vi "TDMS_Create.vi"(0 "reference in":refnum<class "TDMS.lvclass">, 5 "error in (no error)":errorcluster, 6 "Time Data":refnum<class "GSwFormDSP.lvclass">, 7 "Application Name":string, 9 "State Queue":string[](array[string])) -> (14 "reference out":refnum<class "TDMS.lvclass">, 19 "error out":errorcluster)   [LabVIEW 2022 SP3, in "TDMS.lvclass"]
doc: "Constructor."
uses:
  TDMS.lvclass
  C:/Program Files/National Instruments/LabVIEW 2022/vi.lib/addons/_AddQ/G#Object/G#Object.lvclass
  W:/projects/archives/23 Charette AI Group/SPWB/API/Generic Utilities_class/Generic Utilities.lvclass
  API/GSwFormDSP_class/GSwFormDSP.lvclass
  <vilib>/addons/_AddQ/G#Object/G#Object.lvclass
  API/Generic Utilities_class/Generic Utilities.lvclass
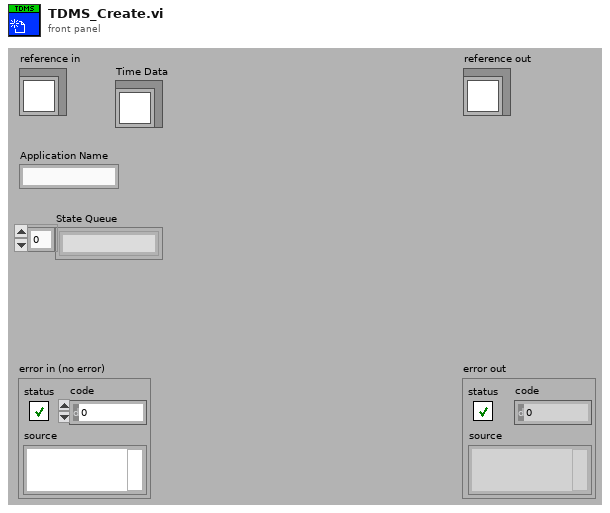
[diagram p1: front panel]
types:
  T1 = typedef "TDMS.lvclass/ObjectAttributesRef.ctl" = refnum<data-value>
  T2 = typedef "TDMS.lvclass/ObjectAttributes.ctl" = cluster{"Time Data":refnum<class "GSwFormDSP.lvclass">, "New Time Data Obj?":bool}
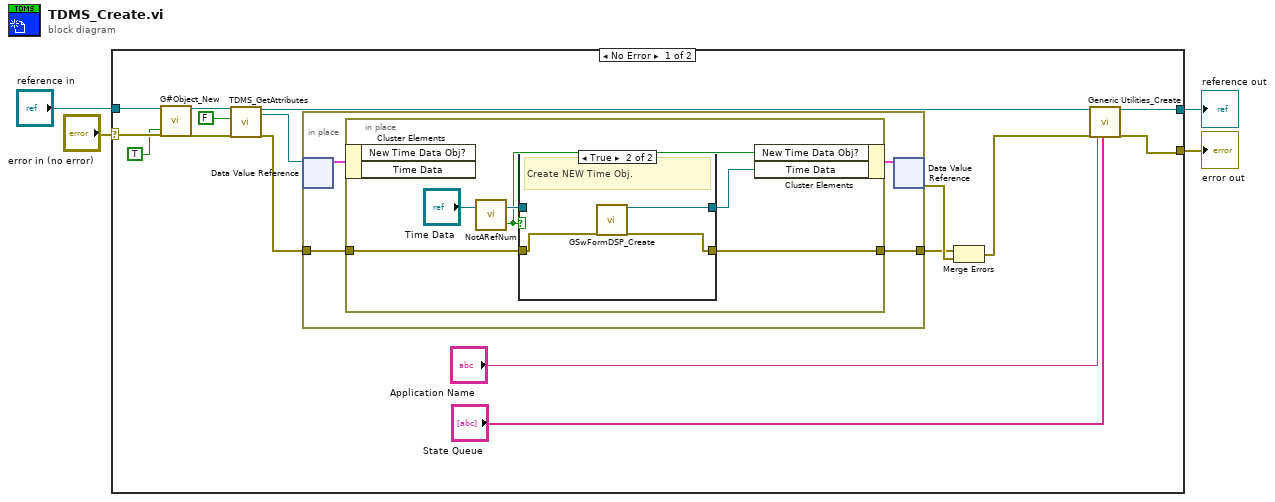
[diagram p0: block diagram]
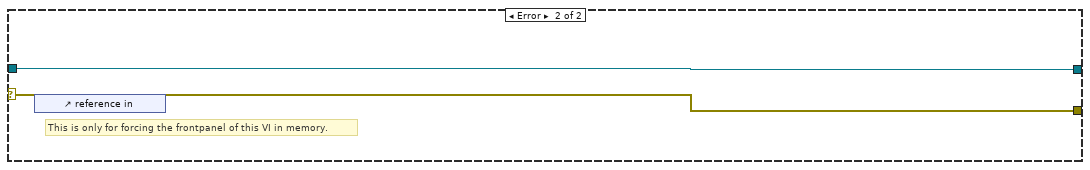
[diagram p3: hidden frame]
diagram:
  n1 = case shown="No Error" "error in (no error)" {
    selector: "error in (no error)" -> [w19 w37]
    tunnel: [w9 w37] -> w3
    tunnel: [w11 w36] -> w1
    tunnel: "reference in" -> [w20 w36]
    frame No Error {
      n2 = call <vilib>:"G#Object_New.vi"("reference in"=w20, "error in (no error)"=w19, "user counter (T)?"=TRUE ("User Counter")) -> ("reference out"=w14:refnum<class "TDMS.lvclass">, "error out"=w13:errorcluster)  [unwired: 14 in, 1 out]
      n3 = call "TDMS_GetAttributes.vi"("reference in"=w14, "return data? (T)"=FALSE ("return data"), "error in (no error)"=w13) -> ("reference out"=w12:refnum<class "TDMS.lvclass">, "attributes ref"=w16:T1, "error out"=w7:errorcluster)  [unwired: 13 in, 1 out]
      n4 = in-place {
        in-place-border: w7 -> [w22]
        in-place-border: [w21] -> w6
        n5 = in-place-dvr #1(w16) -> (w23:T2)  [unwired: 1 out]
        n6 = in-place {
          in-place-border: w22 -> [w27]
          in-place-border: [w26] -> w21
          n7 = in-place-cluster #2(w23) -> ()  [unwired: 2 out]
          n8 = call-dynamic "NotARefNum.vi"("reference in"="Time Data") -> ("not a refnum?"=w25:bool, "reference out"=w30:refnum<class "GSwFormDSP.lvclass">)  [unwired: 1 in]
          n9 = case shown="True" w25 {
            tunnel: [w32 w33] -> w28
            tunnel: w30 -> [w32 _]
            tunnel: w27 -> [w31 w35]
            tunnel: [w31 w34] -> w26
            frame False {
              # "Copy an existing reference."
            }
            frame True {
              # "Create NEW Time Obj."
              n10 = call "GSwFormDSP_Create.vi"("error in (no error)"=w35) -> ("reference out"=w33:refnum<class "GSwFormDSP.lvclass">, "error out"=w34:errorcluster)  [unwired: 17 in]
            }
          }
          n11 = in-place-cluster #2("New Time Data Obj?"=w25, "Time Data"=w28) -> (w24:T2)
        }
        n12 = in-place-dvr #1(w24) -> (w17:errorcluster)  [unwired: 1 out]
      }
      n13 = Merge Errors(w6, w17) -> (w10:errorcluster)
      n14 = call "Generic Utilities_Create.vi"("reference in"=w12, "error in (no error)"=w10, "Application Name"="Application Name", "State Queue"="State Queue") -> ("reference out"=w11:refnum<class "TDMS.lvclass">, "error out"=w9:errorcluster)  [unwired: 14 in]
    }
    frame Error {
      # "This is only for forcing the frontpanel of this VI in memory."
      n15 = control-ref of="reference in"() -> ()  [unwired: 1 out]
    }
  }
  "error out" <- w3
  "reference out" <- w1
